vi "Define connected stages with dialog.vi"(0 "System no.":i32=1 min=1 max=4 step=1, 5 "error in":errorcluster) -> (14 "Stage selection":string[](array[string]), 19 "error out":errorcluster)   [LabVIEW 2020]
doc: "This VI reads the connected axes from Global2.vi and the available stages using VST?.vi and returns the stage names in a ring control. If there are no entries in that ring control, PIStages.dat was not found, or is marked read-only. Run GCSLibrarySetup.exe to register PIStages.dat correctly. In Microsoft Explorer, right-click the file PIStages.dat and select \"Properties\". Make sure that the \"read-only\" attribute is not checked. \nIf OK is pressed, the chosen assignment in Connected stages is written into Stage selection. If Cancel is pressed, the contents of Stage selection are not changed. For axes without a stage connected, choose \"NOSTAGE\".\n\nC-877, C-884, E-871, E-873: VI is valid via USB interface only.\nC-867: VI is valid via RS232 DaisyChain, USB or USB DaisyChain only."
uses:
  General command.llb/Global2 (Array).vi
panel:
  in  "Cancel":bool
  in  "O.k.":bool
  out "Conn. Axes":string[](array[string])
  in  "Connected stages":u16[](array[ring])
  # "This VI reads the connected axes from Global2.vi and the available stages using VST?.vi and returns the stage names in a ring control. If \"O.k.\"\nis pressed, the chosen assignment in \"Connected stages\" is written into \"Stage selection\". If \"Cancel\" is pressed, the contents of \"Stage selection\" are not changed. For axes without a stage connected choose \"NOSTAGE\"."
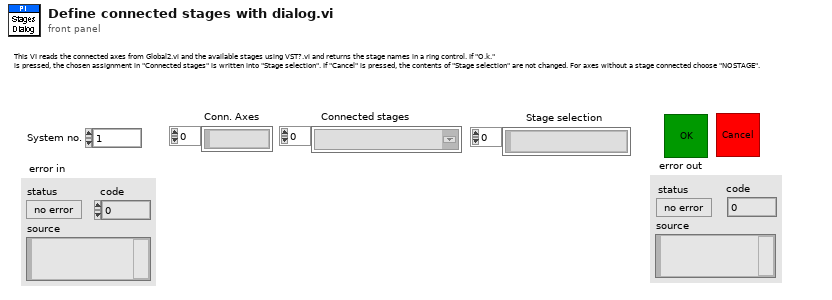
[diagram p1: front panel]
types:
  T1 = typedef "Controller names.ctl" = enum16{"None", "Analog", "C-702", "C-413", "C-414", "C-843", "C-843.PM", "C-844", "C-848", "C-865", "C-866", "C-867", "C-877", "C-880", "C-884", "C-885", "C-886", "C-887", "C-891", "E-135", "E-516", "E-517", "E-518", "E-709", "E-710", "E-712", "E-725", "E-727", "E-753", "E-754", "E-755", "E-761", "E-816", "E-861", "E-870", "E-871", "E-872", "E-873", "E-874", "F-206", "HydraPollux", "M-840", "M-850", "M-8X0", "Mercury", "Mercury_GCS", "PI_GCS2"}
  T2 = cluster{"Conn. axes":string[], "Controller name":T1}[]
  T3 = cluster{"Conn. axes":string[], "Controller name":T1}
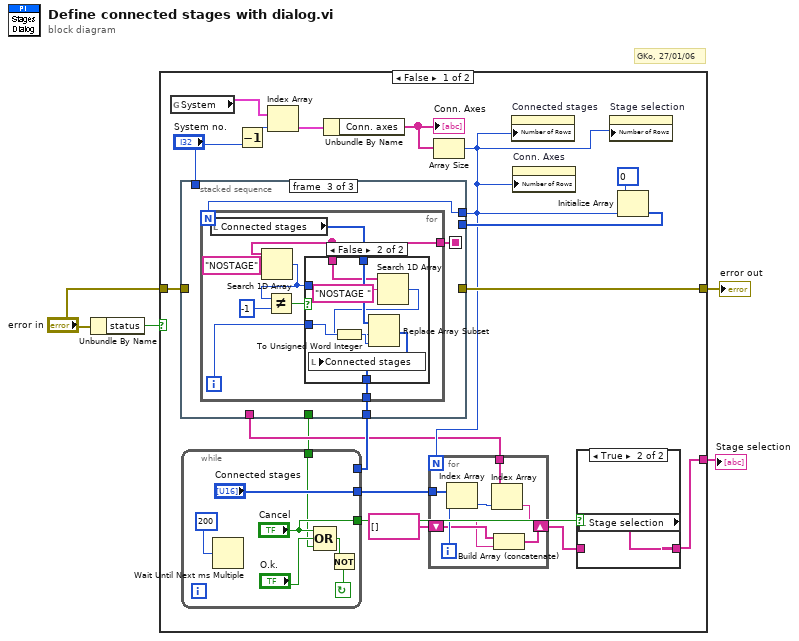
[diagram p0: block diagram]
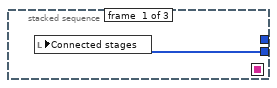
[diagram p2: hidden frame]
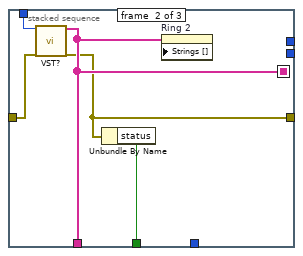
[diagram p3: hidden frame]
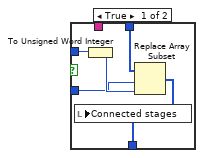
[diagram p4: hidden frame]
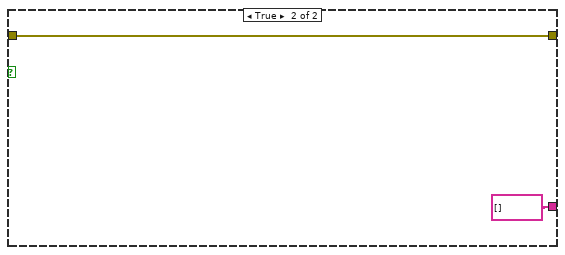
[diagram p6: hidden frame]
diagram:
  # "GKo, 27/01/06"
  n1 = Unbundle By Name("error in") -> ("status"=w3:bool)
  n2 = case shown="False" w3 {
    tunnel: [w17 w69] -> w2
    tunnel: "error in" -> [w22 w69]
    tunnel: [w15 string[] [] ("Stage selection")] -> w1
    frame False {
      w14 = u16 0 items=[""] ("Ring")
      n3 = global read "Global2 (Array).vi" "System"() -> (w9:T2)
      n4 = Decrement(x="System no.") -> (x-1=w7:i32)
      n5 = Index Array(array=w9, index=w7) -> (element=w6:T3)
      n6 = Unbundle By Name(w6) -> ("Conn. axes"=w5:string[])
      "Conn. Axes" <- w5
      n7 = Array Size(array=w5) -> (size(s)=w13:i32)
      n8 = property on="Connected stages" class="Arr (strict)"("Number of Rows"=w13) -> ()  [unwired: 2 in, 2 out]
      n9 = property on="Conn. Axes" class="Arr (strict)"("Number of Rows"=w13) -> ()  [unwired: 2 in, 2 out]
      n10 = property on="Stage selection" class="Arr (strict)"("Number of Rows"=w13) -> ()  [unwired: 2 in, 2 out]
      n11 = Initialize Array(w14, w13) -> (w18:u16[])
      n12 = stacked-sequence {
        seq-local: [_ w33 _] -> [_ _ w36]
        tunnel: w22 -> [_ w35 _]
        tunnel: "System no." -> [_ w34 _]
        tunnel: [_ w32 _] -> w17
        tunnel: [_ w33 _] -> w11
        tunnel: w18 -> [w30 _ _]
        tunnel: w13 -> [_ _ w38]
        tunnel: [_ _ w37] -> w12
        tunnel: [_ w31 _] -> w10
        frame #0 {
          n13 = local write "Connected stages"(w30) -> ()
        }
        frame #1 {
          n14 = call "VST?.vi"("System no."=w34, "error in"=w35) -> ("Available stages"=w33:string[], "error out"=w32:errorcluster)  [unwired: 16 out]
          n15 = Unbundle By Name(w32) -> ("status"=w31:bool)
          n16 = property on="Ring 2" class="Ring (strict)"("Strings []"=w33) -> ()  [unwired: 2 in, 2 out]
        }
        frame #2 {
          n17 = for {
            N: w38 -> [_]
            tunnel: [w43] -> w37
            tunnel: w36 -> [w39]
            i -> [w44]
            n18 = local read "Connected stages"() -> (w45:u16[])
            n19 = Search 1D Array(1D array=w39, element="NOSTAGE") -> (index of element=w42:i32)  [unwired: 1 out]
            n20 = Not Equal?(x=w42, y=-1) -> (x != y?=w40:bool)
            n21 = case shown="False" w40 {
              tunnel: w45 -> [w51 w58]
              tunnel: w42 -> [w50 _]
              tunnel: w44 -> [w48 w56]
              tunnel: [w47 w55] -> w43
              tunnel: w39 -> [_ w54]
              frame True {
                n22 = To Unsigned Word Integer(number=w50) -> (unsigned 16bit integer=w49:u16)
                n23 = Replace Array Subset(array=w51, new element=w49, index=w48) -> (w47:u16[])
                n24 = local write "Connected stages"(w47) -> ()
              }
              frame False {
                n25 = Search 1D Array(1D array=w54, element="NOSTAGE ") -> (index of element=w53:i32)  [unwired: 1 out]
                n26 = To Unsigned Word Integer(number=w53) -> (unsigned 16bit integer=w57:u16)
                n27 = Replace Array Subset(array=w58, new element=w57, index=w56) -> (w55:u16[])
                n28 = local write "Connected stages"(w55) -> ()
              }
            }
          }
        }
      }
      n29 = while {
        tunnel: w10 -> [w23]
        tunnel: w12 -> [_]
        tunnel: ["Connected stages"] -> w19
        tunnel: ["Cancel"] -> w21
        stop <- w26 continue-if-true
        n30 = Wait Until Next ms Multiple(millisecond multiple=u32 200) -> ()  [unwired: 1 out]
        n31 = Compound Arithmetic op=OR("Cancel", "O.k.", w23) -> (w27:bool)
        n32 = Not(x=w27) -> (.not. x?=w26:bool)
      }
      n33 = for {
        N: w13 -> [_]
        tunnel: w19 -> [w64]
        tunnel: w11 -> [w63]
        shift-right: [w59] -> w16
        shift-left: string[] [] -> [w61]
        i -> [w65]
        n34 = Index Array(array=w64, index=w65) -> (element=w62:u16)
        n35 = Index Array(array=w63, index=w62) -> (element=w60:string)
        n36 = Build Array (concatenate)(w61, w60) -> (w59:string[])
      }
      n37 = case shown="True" w21 {
        tunnel: w16 -> [w66 _]
        tunnel: [w66 w67] -> w15
        frame False {
        }
        frame True {
          n38 = local read "Stage selection"() -> (w67:string[])
        }
      }
    }
    frame True {
    }
  }
  "error out" <- w2
  "Stage selection" <- w1
